vi "BuildCommandString.vi"(3 "error in":errorcluster, 4 "Numeric Value":i32, 5 "Command":string) -> (0 "error out":errorcluster, 2 "Result":string)   [LabVIEW 2023]
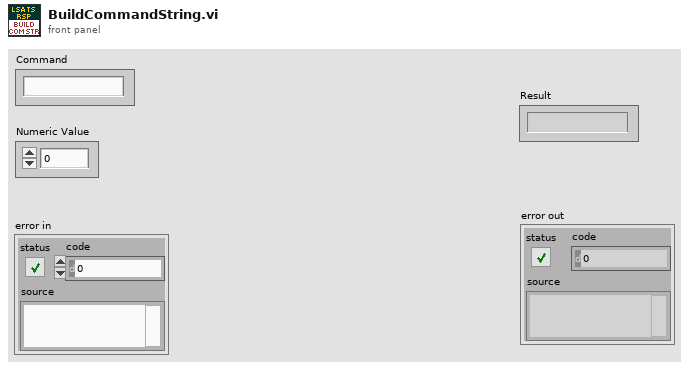
[diagram p1: front panel]
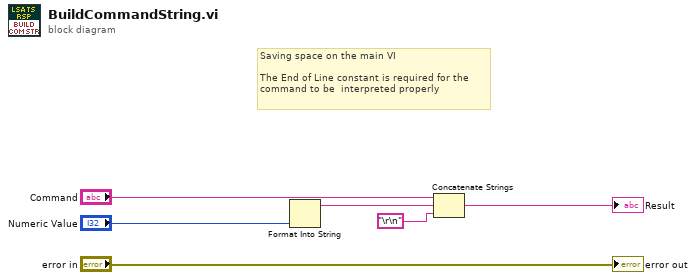
[diagram p0: block diagram]
diagram:
  # "Saving space on the main VI\n\nThe End of Line constant is required for the \ncommand to be  interpreted properly"
  n1 = Format Into String("Numeric Value") -> (resulting string=w2:string)  [unwired: 3 in, 1 out]
  n2 = Concatenate Strings("Command", w2, "\r\n") -> (→"Result":string)
  "error out" <- "error in"
